vi "RichToFlatrfcontrol_StopGPSPollResponse.vi"(5 "OutputClusterType":T1, 11 "InputCluster":T2) -> (3 "OutputCluster":T1)   [LabVIEW 2024, in "FlexSDR_gRPC_client.lvlib"]
uses:
  rfcontrol_StopGPSPollResponse.ctl
  rfcontrol_StopGPSPollResponse_Flat.ctl
  FlexSDR_gRPC_client.lvlib
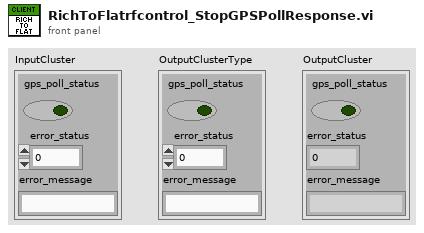
[diagram p1: front panel]
types:
  T1 = typedef "FlexSDR_gRPC_client.lvlib/rfcontrol_StopGPSPollResponse_Flat.ctl" = cluster{"gps_poll_status":bool, "error_status":i32, "error_message":string}
  T2 = typedef "FlexSDR_gRPC_client.lvlib/rfcontrol_StopGPSPollResponse.ctl" = cluster{"gps_poll_status":bool, "error_status":i32, "error_message":string}
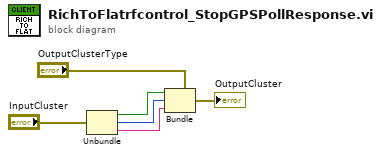
[diagram p0: block diagram]
diagram:
  n1 = Unbundle "Unbundle"("InputCluster") -> ("gps_poll_status"=w3:bool, "error_status"=w2:i32, "error_message"=w1:string)
  n2 = Bundle "Bundle"(cluster="OutputClusterType", "gps_poll_status"=w3, "error_status"=w2, "error_message"=w1) -> (→"OutputCluster":T1)
